vi "Initialize.vi"(8 "error in (no error)":errorcluster, 10 "Reset?":bool, 11 "Fluke Calibrator in":refnum<class "Fluke Calibrator.lvclass">) -> (0 "error out":errorcluster, 3 "Fluke Calibrator out":refnum<class "Fluke Calibrator.lvclass">)   [LabVIEW 2023, in "Fluke Calibrator.lvclass"]
uses:
  Fluke Calibrator.lvclass
  Fluke Calibrator.lvclass/Fluke Calibrator.ctl
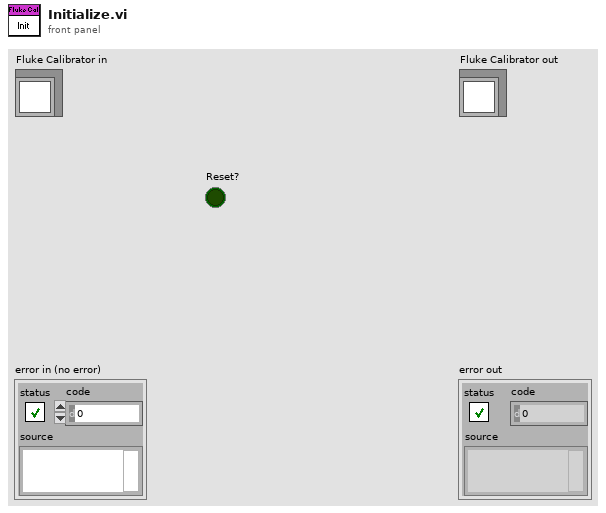
[diagram p1: front panel]
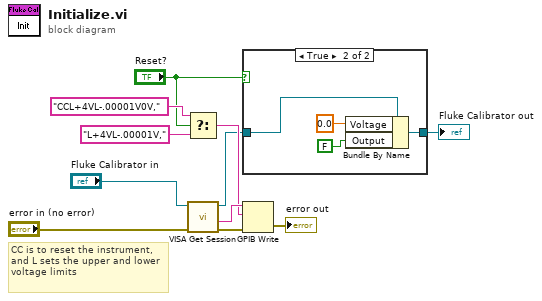
[diagram p0: block diagram]
diagram:
  # "CC is to reset the instrument, and L sets the upper and lower voltage limits"
  n1 = Select(t="CCL+4VL-.00001V0V," ("data"), s="Reset?", f="L+4VL-.00001V," ("data")) -> (s? t:f=w4:string)
  n2 = call-dynamic "VISA Get Session.vi"("error in (no error)"="error in (no error)", "Instrument.lvclass in"="Fluke Calibrator in") -> ("error out"=w8:errorcluster, "GPIB string"=w9:string, "Instrument.lvclass out"=w3:refnum<class "Fluke Calibrator.lvclass">)  [unwired: 6 in, 1 out]
  n3 = case shown="True" "Reset?" {
    tunnel: w3 -> [w12 w16]
    tunnel: [w12 w15] -> w1
    frame False {
    }
    frame True {
      n4 = Bundle By Name(cluster=w16, "Voltage"=0.0, "Output"=FALSE) -> (w15:refnum<class "Fluke Calibrator.lvclass">)
    }
  }
  "Fluke Calibrator out" <- w1
  n5 = GPIB Write(0:w9, 1:w4, 3:w8) -> (6:→"error out":errorcluster)  [unwired: 2 in, 1 out]
